vi "find xy cut positions (subVI).vi"(9 "r":dbl, 10 "input frame":u16[][](array[numeric]), 11 "Nx":dbl) -> (2 "projection profiles":u32[](array[numeric]), 3 "xy cut positions":dbl[](array[numeric]))   [LabVIEW 2024]
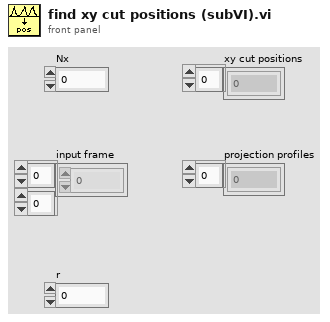
[diagram p1: front panel]
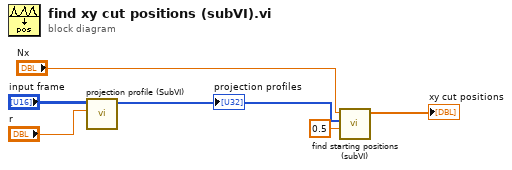
[diagram p0: block diagram]
diagram:
  n1 = call "projection profile (SubVI).vi"("r"="r", "input frame"="input frame") -> ("Array"=w4:u32[])  [unwired: 9 in]
  "projection profiles" <- w4
  n2 = call "find starting positions (subVI).vi"("threshold level [0-1]"=0.5, "proj profile"=w4, "Nx"="Nx") -> ("starting positions"=→"xy cut positions":dbl[])  [unwired: 8 in]
